vi "NI6008 Status Report.vi"(8 "error in (no error)":errorcluster, 10 "Data":T1, 11 "I_NI6008 in":refnum<class "I_NI6008.lvclass">) -> (0 "error out":errorcluster, 3 "I_NI6008 out":refnum<class "I_NI6008.lvclass">)   [LabVIEW 2020, in "Actor_NI6008.lvlib" / "I_NI6008.lvclass"]
uses:
  I_NI6008.lvclass
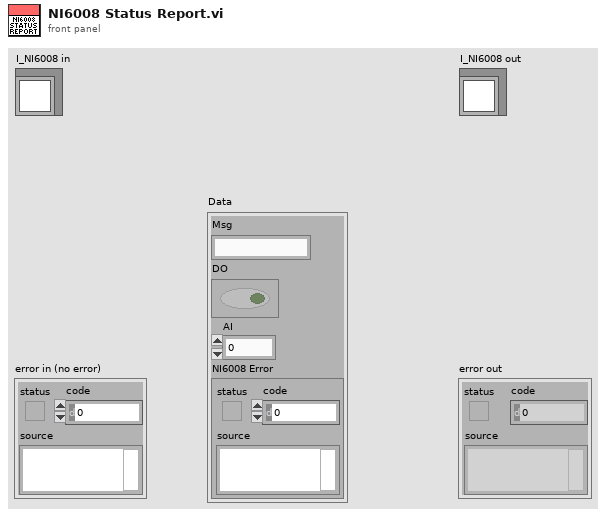
[diagram p1: front panel]
types:
  T1 = cluster{"Msg":string, "DO":bool[], "AI":dbl, "NI6008 Error":errorcluster}
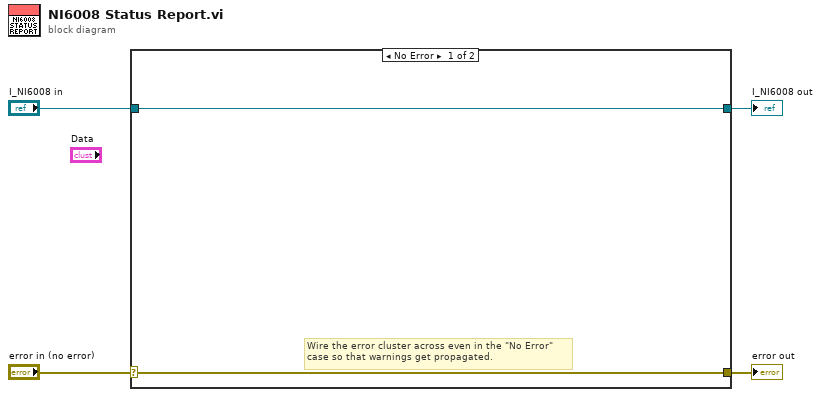
[diagram p0: block diagram]
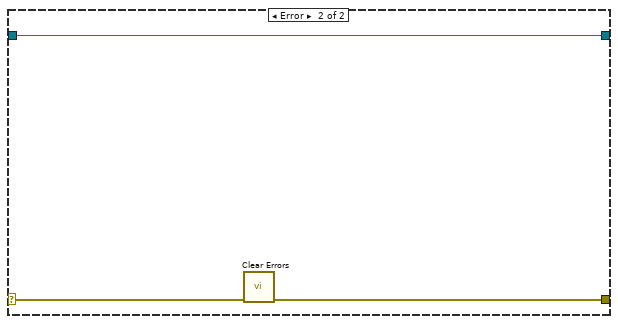
[diagram p2: hidden frame]
diagram:
  n1 = case shown="No Error" "error in (no error)" {
    selector: "error in (no error)" -> [w5 w8]
    tunnel: [w5 w7] -> w3
    tunnel: [w6 w9] -> w1
    tunnel: "I_NI6008 in" -> [w6 w9]
    frame No Error {
      # "Wire the error cluster across even in the \"No Error\"\ncase so that warnings get propagated."
    }
    frame Error {
      n2 = call <vilib>:"Clear Errors.vi"("error in (no error)"=w8) -> ("error out"=w7:errorcluster)  [unwired: 5 in, 1 out]
    }
  }
  "error out" <- w3
  "I_NI6008 out" <- w1
